vi "Service Stop Handler.vi"(8 "error in (no error)":errorcluster, 9 "Stop Server User Event":T1, 10 "Stop Button [ref]":refnum<vi>, 11 "MeasurementServiceV2 in":refnum<class "Measurement Service V2.lvclass">) -> (0 "error out":errorcluster, 3 "MeasurementServiceV2 out":refnum<class "Measurement Service V2.lvclass">)   [LabVIEW 2020, in "MeasurementLink Measurement Server.lvlib" / "Measurement Service V2.lvclass"]
uses:
  Measurement Service V2.lvclass
  Helpers/TypeDefs/Stop Server User Event.ctl
  Measurement Service V2.lvclass/Measurement Service V2.ctl
  MeasurementLink Measurement Service Base V2/RPC Service/MeasurementService/MeasurementServiceBaseV2.lvclass
  C:/Program Files/National Instruments/LabVIEW 2020/vi.lib/gRPC/LabVIEW gRPC Servicer/ServiceBase/ServiceBase.lvclass
  IMeasurement Service/IMeasurement Service.lvclass
  MeasurementLink Measurement Server.lvlib
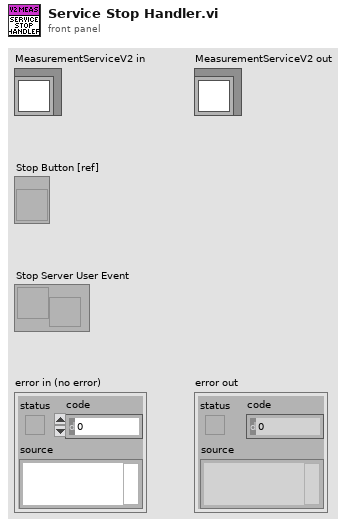
[diagram p1: front panel]
types:
  T1 = typedef "MeasurementLink Measurement Server.lvlib/Stop Server User Event.ctl" = refnum<user-event>
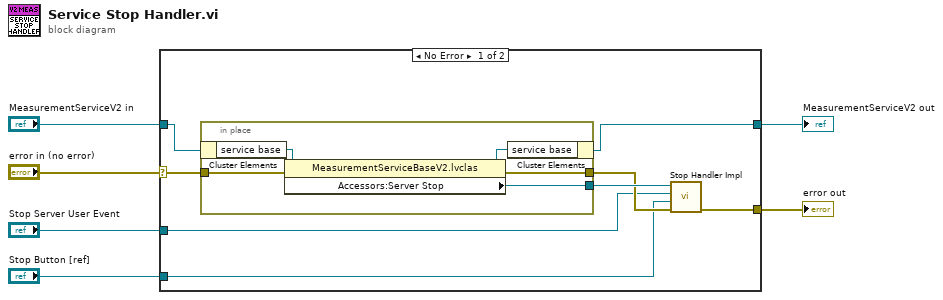
[diagram p0: block diagram]
diagram:
  n1 = case shown="No Error" "error in (no error)" {
    selector: "error in (no error)" -> [w13 w21]
    tunnel: [w12 w21] -> w5
    tunnel: [w11 w20] -> w3
    tunnel: "MeasurementServiceV2 in" -> [w14 w20]
    tunnel: "Stop Button [ref]" -> [w8 _]
    tunnel: "Stop Server User Event" -> [w7 _]
    frame No Error {
      n2 = in-place {
        in-place-border: [w17] -> w10
        in-place-border: w13 -> [w16]
        in-place-border: [w15] -> w9
        n3 = in-place-cluster #1(w14) -> ("service base"=w19:refnum<class "MeasurementServiceBaseV2.lvclass">)
        n4 = property class="MeasurementServiceBaseV2.lvclas"(reference=w19, error in=w16) -> (reference out=w18:refnum<class "MeasurementServiceBaseV2.lvclass">, error out=w15:errorcluster, "Accessors:Server Stop"=w17:refnum<user-event>)
        n5 = in-place-cluster #1("service base"=w18) -> (w11:refnum<class "Measurement Service V2.lvclass">)
      }
      n6 = call "Stop Handler Impl.vi"("error in (no error)"=w9, "Stop Button [ref]"=w8, "Stop Server User Event"=w7, "Stop Server Broadcast Event"=w10) -> ("error out"=w12:errorcluster)  [unwired: 7 in]
    }
    frame Error {
    }
  }
  "error out" <- w5
  "MeasurementServiceV2 out" <- w3
